vi "JL_Heat_Set Up.vi"(8 "error in (no error)":errorcluster, 9 "GEA Inputs":T1 {"Destination" format="%.0x"; "Source" format="%.0x"}, 11 ".NET Refnum in":refnum<k24>) -> (0 "error out":errorcluster, 3 "ERD Data Out":T2[](array[typedef]) {"ERD Number" format="%.0x"})   [LabVIEW 2016]
uses:
  Common/LabVIEW GEA2 Toolkit/LabVIEW_GEA2_Toolkit.lvlibp/type defs/ERD Read Data Out.ctl
  Common/LabVIEW GEA2 Toolkit/LabVIEW_GEA2_Toolkit.lvlibp/type defs/Source_Destination.ctl
  Q:/Common/DLLs/GEA3/GeaCommunication.dll
  Common/DLLs/GEA3/GeaCommunication.dll
  Common/LabVIEW GEA2 Toolkit/LabVIEW_GEA2_Toolkit.lvlibp/type defs/ERD Read Data In.ctl
  Common/LabVIEW GEA2 Toolkit/LabVIEW_GEA2_Toolkit.lvlibp/type defs/Data Type.ctl
  Common/LabVIEW GEA2 Toolkit/LabVIEW_GEA2_Toolkit.lvlibp
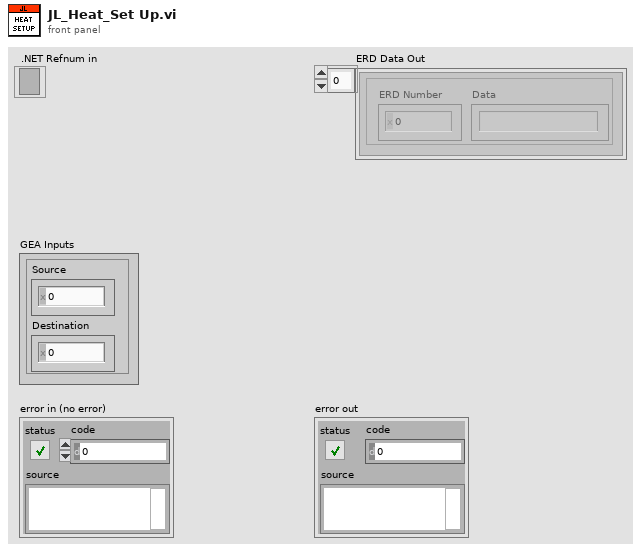
[diagram p1: front panel]
types:
  T1 = typedef "LabVIEW_GEA2_Toolkit.lvlibp/Source_Destination.ctl" = cluster{"Source":u8, "Destination":u8}
  T2 = typedef "LabVIEW_GEA2_Toolkit.lvlibp/ERD Read Data Out.ctl" = cluster{"ERD Number":u16, "Data":string}
  T3 = typedef "LabVIEW_GEA2_Toolkit.lvlibp/ERD Read Data In.ctl" = cluster{"ERD Number":u16, "Data Type":T4}
  T4 = typedef "LabVIEW_GEA2_Toolkit.lvlibp/Data Type.ctl" = enum16{"string", "boolean", "uint8_t", "uint16_t", "uint32_t", "uint64_t", "int8_t", "int16_t", "int32_t", "int64_t"}
  T5 = cluster{"Erd Numbers":u16[], "Erd Names":string[]}
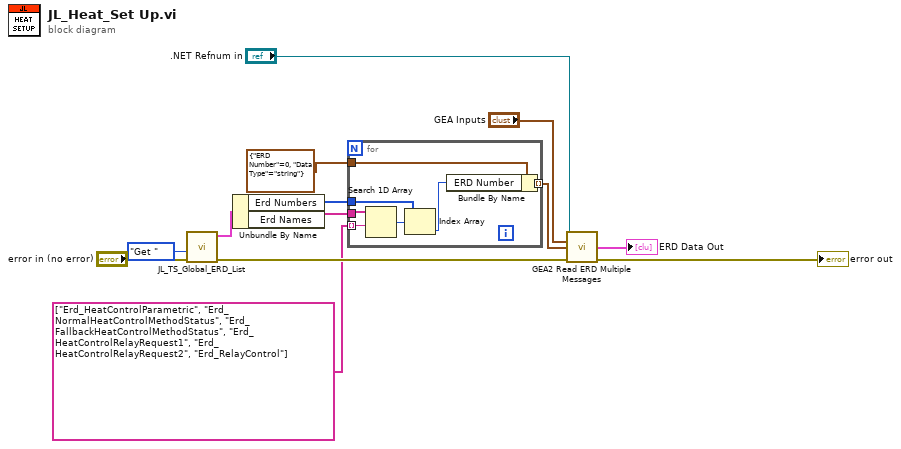
[diagram p0: block diagram]
diagram:
  n1 = call "JL_TS_Global_ERD_List.vi"("Error In"="error in (no error)", "Action"=enum16{"Set", "Get "}."Get ") -> ("Error Out"=w12:errorcluster, "TS ERD Names Number"=w6:T5)  [unwired: 8 in]
  n2 = Unbundle By Name(w6) -> ("Erd Numbers"=w3:u16[], "Erd Names"=w5:string[])
  n3 = for {
    tunnel: w5 -> [w20]
    tunnel: string[] ["Erd_HeatControlParametric", "Erd_NormalHeatControlMethodStatus", "Erd_FallbackHeatControlMethodStatus", "Erd_HeatControlRelayRequest1", "Erd_HeatControlRelayRequest2", "Erd_RelayControl"] -> [w19] mode=indexing
    tunnel: w3 -> [w17]
    tunnel: T3 {"ERD Number"=0, "Data Type"=enum."string"} ("ERD Read Data In") -> [w16]
    tunnel: [w14] -> w1 mode=indexing
    n4 = Search 1D Array(1D array=w20, element=w19) -> (index of element=w18:i32)  [unwired: 1 in]
    n5 = Index Array(array=w17, index=w18) -> (element=w15:u16)
    n6 = Bundle By Name(cluster=w16, "ERD Number"=w15) -> (w14:T3)
  }
  n7 = call "GEA2 Read ERD Multiple Messages.vi"("GEA2 Reference In"=".NET Refnum in", "GEA Inputs"="GEA Inputs", "Read ERD List"=w1, "Error In"=w12) -> ("ERD Data Out"=→"ERD Data Out":T2[], "Error Out"=→"error out":errorcluster)  [unwired: 8 in, 2 out]
